vi "Vector_flip_y.vi"(11 "x,y":cluster{"X ":i16, "Y ":i16}) -> (3 "x,-y":cluster{"X ":i16, "Y ":i16})   [LabVIEW 2024]
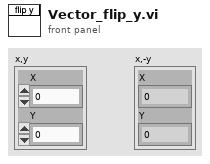
[diagram p1: front panel]
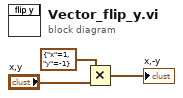
[diagram p0: block diagram]
diagram:
  n1 = Multiply(x=cluster{"x":i16, "y":i16} {"x"=1, "y"=-1} ("vector"), y="x,y") -> (x*y=→"x,-y":cluster{i16, i16})
